vi "CalculateDelay_2chan_16_2.vi"(8 "input valid":bool=TRUE, 9 "cos_fi":fxp<+/-,16,2>, 10 "sin fi":fxp<+/-,16,2>, 11 "Data in":fxp<+/-,16,14>[](array[numeric])=[0.0, 0.0, 0.0, 0.0]) -> (0 "output valid":bool, 3 "Data out":fxp<+/-,16,14>[](array[numeric]))   [LabVIEW 2013]
doc: "Calculates various combinations on I_in, Q_in and cos(fi) and sin(fi) to be used later to delay the output signal"
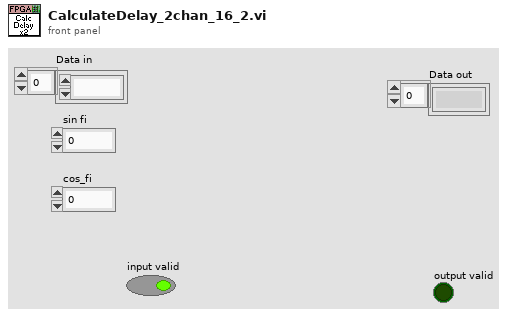
[diagram p1: front panel]
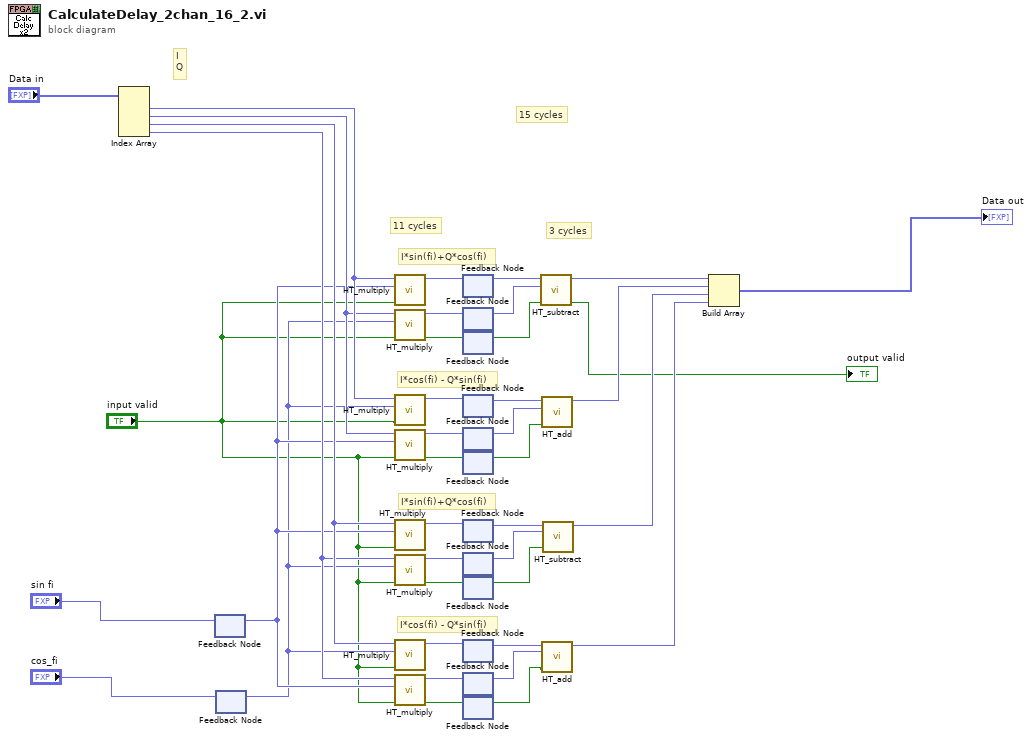
[diagram p0: block diagram]
diagram:
  # "3 cycles"
  # "11 cycles"
  # "15 cycles"
  # "I*cos(fi) - Q*sin(fi)"
  # "I*sin(fi)+Q*cos(fi)"
  # "I*cos(fi) - Q*sin(fi)"
  # "I\nQ"
  # "I*sin(fi)+Q*cos(fi)"
  n1 = Index Array(array="Data in") -> (element #1=w33:fxp<+/-,16,14>, element #2=w32:fxp<+/-,16,14>, element #3=w24:fxp<+/-,16,14>, element #4=w23:fxp<+/-,16,14>)  [unwired: 4 in]
  n2 = feedback #1() -> (w22:fxp<+/-,16,2>)  [unwired: 1 in]
  n3 = feedback-in #1("sin fi") -> ()
  n4 = feedback #2() -> (w21:fxp<+/-,16,2>)  [unwired: 1 in]
  n5 = feedback-in #2("cos_fi") -> ()
  n6 = call "HT_multiply.vi"("input valid"="input valid", "y"=w22, "x"=w33) -> ("x*y"=w39:fxp<+/-,16,14>)  [unwired: 7 in, 1 out]
  n7 = call "HT_multiply.vi"("input valid"="input valid", "y"=w21, "x"=w32) -> ("output valid"=w37:bool, "x*y"=w38:fxp<+/-,16,14>)  [unwired: 7 in]
  n8 = call "HT_multiply.vi"("input valid"="input valid", "y"=w21, "x"=w33) -> ("x*y"=w34:fxp<+/-,16,14>)  [unwired: 7 in, 1 out]
  n9 = call "HT_multiply.vi"("input valid"="input valid", "y"=w22, "x"=w32) -> ("output valid"=w36:bool, "x*y"=w35:fxp<+/-,16,14>)  [unwired: 7 in]
  n10 = call "HT_multiply.vi"("input valid"="input valid", "y"=w22, "x"=w24) -> ("x*y"=w25:fxp<+/-,16,14>)  [unwired: 7 in, 1 out]
  n11 = call "HT_multiply.vi"("input valid"="input valid", "y"=w21, "x"=w23) -> ("output valid"=w27:bool, "x*y"=w26:fxp<+/-,16,14>)  [unwired: 7 in]
  n12 = call "HT_multiply.vi"("input valid"="input valid", "y"=w21, "x"=w24) -> ("x*y"=w30:fxp<+/-,16,14>)  [unwired: 7 in, 1 out]
  n13 = call "HT_multiply.vi"("input valid"="input valid", "y"=w22, "x"=w23) -> ("output valid"=w28:bool, "x*y"=w29:fxp<+/-,16,14>)  [unwired: 7 in]
  n14 = feedback #3() -> (w5:fxp<+/-,16,14>)  [unwired: 1 in]
  n15 = feedback-in #3(w39) -> ()
  n16 = feedback #4() -> (w1:fxp<+/-,16,14>)  [unwired: 1 in]
  n17 = feedback-in #4(w38) -> ()
  n18 = feedback #5() -> (w2:bool)  [unwired: 1 in]
  n19 = feedback-in #5(w37) -> ()
  n20 = feedback #6() -> (w7:fxp<+/-,16,14>)  [unwired: 1 in]
  n21 = feedback-in #6(w34) -> ()
  n22 = feedback #7() -> (w8:fxp<+/-,16,14>)  [unwired: 1 in]
  n23 = feedback-in #7(w35) -> ()
  n24 = feedback #8() -> (w9:bool)  [unwired: 1 in]
  n25 = feedback-in #8(w36) -> ()
  n26 = feedback #9() -> (w12:fxp<+/-,16,14>)  [unwired: 1 in]
  n27 = feedback-in #9(w25) -> ()
  n28 = feedback #10() -> (w11:fxp<+/-,16,14>)  [unwired: 1 in]
  n29 = feedback-in #10(w26) -> ()
  n30 = feedback #11() -> (w10:bool)  [unwired: 1 in]
  n31 = feedback-in #11(w27) -> ()
  n32 = feedback #12() -> (w17:fxp<+/-,16,14>)  [unwired: 1 in]
  n33 = feedback-in #12(w30) -> ()
  n34 = feedback #13() -> (w16:fxp<+/-,16,14>)  [unwired: 1 in]
  n35 = feedback-in #13(w29) -> ()
  n36 = feedback #14() -> (w15:bool)  [unwired: 1 in]
  n37 = feedback-in #14(w28) -> ()
  n38 = call "HT_subtract.vi"("input valid"=w2, "y"=w1, "x"=w5) -> ("output valid"=→"output valid":bool, "x+y"=w4:fxp<+/-,16,14>)  [unwired: 7 in]
  n39 = call "HT_add.vi"("input valid"=w9, "y"=w8, "x"=w7) -> ("x+y"=w6:fxp<+/-,16,14>)  [unwired: 7 in, 1 out]
  n40 = call "HT_add.vi"("input valid"=w15, "y"=w16, "x"=w17) -> ("x+y"=w14:fxp<+/-,16,14>)  [unwired: 7 in, 1 out]
  n41 = call "HT_subtract.vi"("input valid"=w10, "y"=w11, "x"=w12) -> ("x+y"=w13:fxp<+/-,16,14>)  [unwired: 7 in, 1 out]
  n42 = Build Array(w4, w6, w13, w14) -> (→"Data out":fxp<+/-,16,14>[])
